vi "Get board layout.vi"(11 "Board in":refnum<class "Board.lvclass">) -> (2 "Board layout":cluster{"Occupied":bool, "Piece":T1}[][](array[cluster]), 3 "Board out":refnum<class "Board.lvclass">)   [LabVIEW 2016, in "Chesslib.lvlib" / "Board.lvclass"]
uses:
  Board.lvclass
  typedef/Piece.ctl
  typedef/Color.ctl
  typedef/Piece type.ctl
  typedef/Square.ctl
  typedef/File.ctl
  typedef/Rank.ctl
  Pieces/Piece/Piece.lvclass/Piece.ctl
  Pieces/Piece/Piece.lvclass
  Chesslib.lvlib
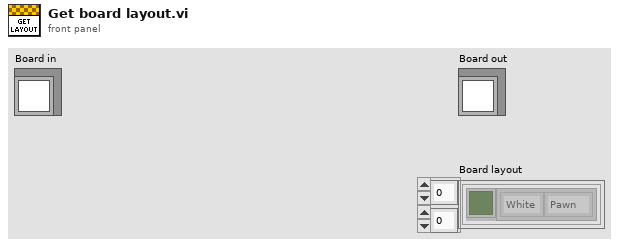
[diagram p1: front panel]
types:
  T1 = typedef "Chesslib.lvlib/Piece.ctl" = cluster{"Color":T2, "Type":T3}
  T2 = typedef "Chesslib.lvlib/Color.ctl" = enum16{"White", "Black"}
  T3 = typedef "Chesslib.lvlib/Piece type.ctl" = enum16{"Pawn", "Bishop", "Knight", "Rook", "Queen", "King"}
  T4 = typedef "Chesslib.lvlib/Square.ctl" = cluster{"File":T5, "Rank":T6}
  T5 = typedef "Chesslib.lvlib/File.ctl" = enum8{"a", "b", "c", "d", "e", "f", "g", "h"}
  T6 = typedef "Chesslib.lvlib/Rank.ctl" = enum8{"1", "2", "3", "4", "5", "6", "7", "8"}
  T7 = cluster{"Occupied":bool, cluster{"Color":T2, "Piece type":T3}}
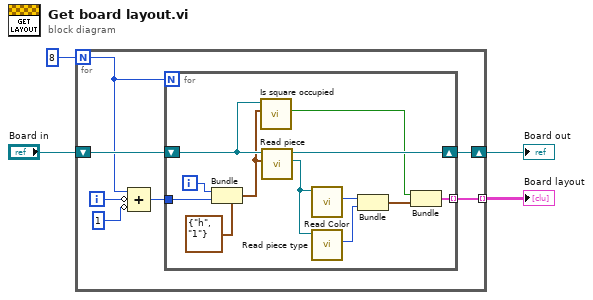
[diagram p0: block diagram]
diagram:
  n1 = for {
    N: 8 -> [w7]
    shift-right: [w10] -> w2
    shift-left: "Board in" -> [w11]
    tunnel: [w9] -> w1 mode=indexing
    i -> [w8]
    n2 = Compound Arithmetic op=ADD(w7, invert w8, invert 1 ("value")) -> (w6:i32)
    n3 = for {
      N: w7 -> [_]
      shift-right: [w23] -> w10
      shift-left: w11 -> [w14]
      tunnel: w6 -> [w18]
      tunnel: [w19] -> w9 mode=indexing
      i -> [w17]
      n4 = Bundle(cluster=T4 {"File"=enum."h", "Rank"=enum."1"} ("Square"), "File"=w17, "Rank"=w18) -> (w12:T4)
      n5 = call "Is square occupied.vi"("Square"=w12, "Board in"=w14) -> ("Occupied"=w13:bool)  [unwired: 7 in, 2 out]
      n6 = call "Read piece.vi"("Square"=w12, "Board in"=w14) -> ("Piece"=w15:refnum<class "Piece.lvclass">, "Board out"=w23:refnum<class "Board.lvclass">)  [unwired: 7 in, 1 out]
      n7 = call "Read Color.vi"("Piece in"=w15) -> ("Color"=w21:T2)  [unwired: 10 in]
      n8 = call-dynamic "Read piece type.vi"("Piece in"=w15) -> ("Piece type"=w22:T3)  [unwired: 10 in]
      n9 = Bundle("Color"=w21, "Piece type"=w22) -> (w20:cluster{"Color":T2, "Piece type":T3})  [unwired: 1 in]
      n10 = Bundle("Occupied"=w13, w20) -> (w19:T7)  [unwired: 1 in]
    }
  }
  "Board out" <- w2
  "Board layout" <- w1
